vi "Combine TDMS Files Into One.vi"(8 "error in (no error)":errorcluster, 10 "TDMS Files":path[](array[path]), 11 "Combined TDMS Path":path) -> (0 "error out":errorcluster, 3 "Success":bool)   [LabVIEW 2015]
doc: "This VI will combine several <B>TDMS Files</B> into a single <B>Combined TDMS Path</B>. If the combine operation performed a successful copy then the <b>Success?</b> will be <b>TRUE</b>. Note that this simply means the merge was successful, it does not mean the output is valid.\n\n-----\nBrian Hoover (Hooovahh)"
uses:
  <vilib>/dlg_ctls.llb/Space Constant.vi
  <vilib>/Platform/system.llb/System Exec.vi
  <vilib>/Utility/error.llb/Trim Whitespace.vi
  <vilib>/Utility/error.llb/Error Cluster From Error Code.vi
  <vilib>/ErrorRing/Error Ring.xnode
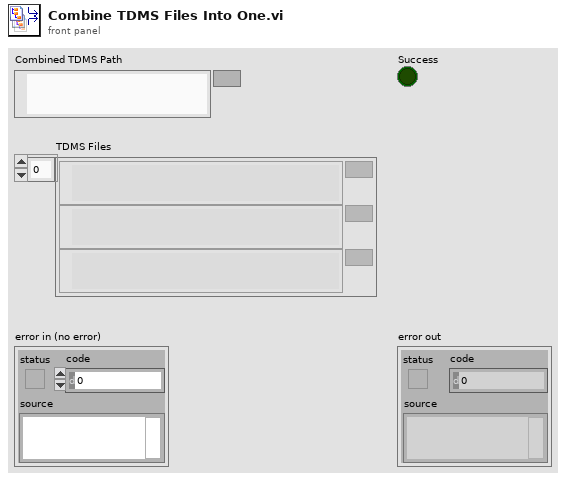
[diagram p1: front panel]
types:
  T1 = enum16{"open", "replace", "create", "open or create", "replace or create", "replace or create with confirmation"}
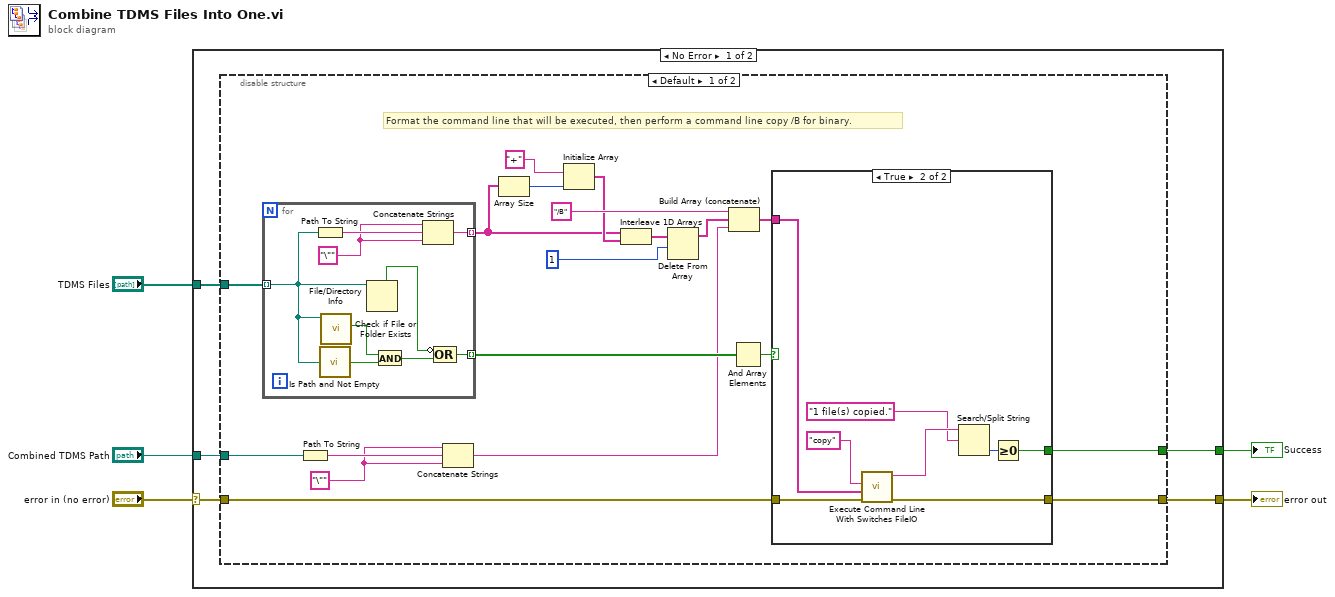
[diagram p0: block diagram]
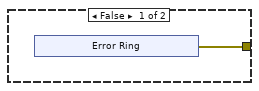
[diagram p2: hidden frame]
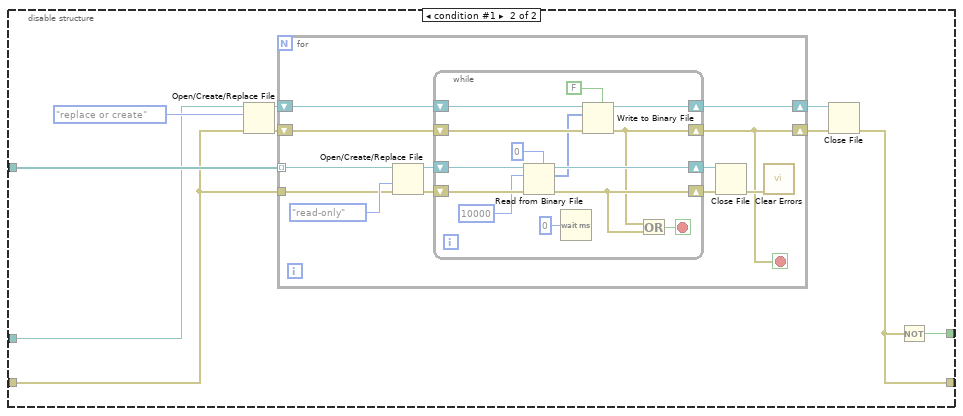
[diagram p3: hidden frame]
diagram:
  n1 = case shown="No Error" "error in (no error)" {
    selector: "error in (no error)" -> [w7 w89]
    tunnel: [w10 w89] -> w5
    tunnel: "TDMS Files" -> [w9 _]
    tunnel: "Combined TDMS Path" -> [w8 _]
    tunnel: [w6 _] -> w1
    frame No Error {
      n2 = disable-structure shown="Default" {
        disable-tunnel: [w29 w55] -> w10
        disable-tunnel: w9 -> [w28 w57]
        disable-tunnel: w8 -> [w26 w56]
        disable-tunnel: w7 -> [w21 w53]
        disable-tunnel: [w11 w54] -> w6
        frame condition #0 (active) {
          w12 = "\"" ("string")
          # "Format the command line that will be executed, then perform a command line copy /B for binary."
          n3 = for {
            tunnel: w28 -> [w45] mode=indexing
            tunnel: [w50] -> w18 mode=indexing
            tunnel: [w51] -> w23 mode=indexing
            w49 = "\"" ("string")
            n4 = Path To String(path=w45) -> (string=w52:string)
            n5 = call <vilib>:"Is Path and Not Empty.vi"("path"=w45) -> ("Is Path and Not Empty?"=w47:bool)  [unwired: 4 in]
            n6 = call <vilib>:"Check if File or Folder Exists.vi"("path"=w45) -> ("file or folder exists?"=w48:bool)  [unwired: 8 in, 2 out]
            n7 = File/Directory Info(path=w45) -> (directory=w44:bool)  [unwired: 1 in, 6 out]
            n8 = And(x=w48, y=w47) -> (x .and. y?=w46:bool)
            n9 = Concatenate Strings(w49, w52, w49) -> (w50:string)
            n10 = Compound Arithmetic op=OR(invert w44, w46) -> (w51:bool)
          }
          n11 = Path To String(path=w26) -> (string=w25:string)
          n12 = Concatenate Strings(w12, w25, w12) -> (w13:string)
          n13 = Array Size(array=w18) -> (size(s)=w17:i32)
          n14 = Initialize Array("+", w17) -> (w19:string[])
          n15 = Interleave 1D Arrays(w18, w19) -> (w16:string[])
          n16 = Delete From Array(array=w16, length=1) -> (array with subset deleted=w15:string[])  [unwired: 1 in, 1 out]
          n17 = Build Array (concatenate)("/B", w15, w13) -> (w24:string[])
          n18 = And Array Elements(Boolean array=w23) -> (logical AND=w22:bool)
          n19 = case shown="True" w22 {
            tunnel: w21 -> [_ w43]
            tunnel: [w30 w42] -> w29
            tunnel: w24 -> [_ w40]
            tunnel: [_ w36] -> w11
            frame False {
              n20 = xnode "Error Ring"() -> ("error out"=w30:errorcluster)
            }
            frame True {
              n21 = call "Execute Command Line With Switches FileIO.vi"("error in (no error)"=w43, "Command Line Switches"=w40, "Command (dir)"="copy") -> ("error out"=w42:errorcluster, "Standard Output"=w39:string)  [unwired: 7 in]
              n22 = Search/Split String(string=w39, search string/char (-)="1 file(s) copied.") -> (offset of match=w37:i32)  [unwired: 1 in, 2 out]
              n23 = Greater Or Equal To 0?(x=w37) -> (x >= 0?=w36:bool)
            }
          }
        }
        frame condition #1 {
          n24 = Open/Create/Replace File(file path (use dialog)=w56, error in=w53, operation (0:open)=T1."replace or create") -> (refnum out=w58:refnum<file>, error out=w60:errorcluster)  [unwired: 3 in, 1 out]
          n25 = for {
            shift-right: [w65] -> w59
            shift-left: w60 -> [w67]
            shift-right: [w74] -> w61
            shift-left: w58 -> [w66]
            tunnel: w57 -> [w64] mode=indexing
            tunnel: w53 -> [w63]
            stop <- w65 stop-if-true
            n26 = Open/Create/Replace File(file path (use dialog)=w64, error in=w63, access (0:read/write)=enum16{"read/write", "read-only", "write-only"}."read-only") -> (refnum out=w73:refnum<file>, error out=w72:errorcluster)  [unwired: 3 in, 1 out]
            n27 = while {
              shift-right: [w86] -> w71
              shift-left: w73 -> [w88]
              shift-right: [w80] -> w70
              shift-left: w72 -> [w87]
              shift-right: [w83] -> w74
              shift-left: w66 -> [w85]
              shift-right: [w78] -> w65
              shift-left: w67 -> [w84]
              stop <- w79 stop-if-true
              n28 = Read from Binary File(5:u8 0, 8:w87, 10:10000 ("count (1)"), 11:w88) -> (0:w80:errorcluster, 2:w82:u8[], 3:w86:refnum<file>)  [unwired: 2 in, 1 out]
              n29 = Wait (ms)(milliseconds to wait=u32 0) -> ()  [unwired: 1 out]
              n30 = Write to Binary File(file (use dialog)=w85, data=w82, error in=w84, 5:FALSE ("prepend array or string size? (T)")) -> (refnum out=w83:refnum<file>, error out=w78:errorcluster)  [unwired: 2 in, 1 out]
              n31 = Or(x=w78, y=w80) -> (x .or. y?=w79:bool)
            }
            n32 = Close File(refnum=w71, error in=w70) -> (error out=w68:errorcluster)  [unwired: 1 out]
            n33 = call <vilib>:"Clear Errors.vi"("error in (no error)"=w68) -> ()  [unwired: 5 in, 2 out]
          }
          n34 = Close File(refnum=w61, error in=w59) -> (error out=w55:errorcluster)  [unwired: 1 out]
          n35 = Not(x=w55) -> (.not. x?=w54:bool)
        }
      }
    }
    frame Error {
    }
  }
  "error out" <- w5
  "Success" <- w1
